vi "varshni fit function.vi"(3 "output control":T1, 4 "data":T2, 5 "X":dbl[](array[numeric]), 6 "a":dbl[](array[numeric])) -> (0 "error out":errorcluster, 1 "f'(X,a)":dbl[][](array[numeric]), 2 "f(X,a)":dbl[](array[numeric]))   [LabVIEW 2010]
doc: "This template is the starting point for creating a model function to be passed to the Nonlinear Curve Fit.vi."
uses:
  <vilib>/gmath/NumericalOptimization/objective function data.ctl
  <vilib>/gmath/NumericalOptimization/LM_output select.ctl
  <vilib>/gmath/NI_Gmath.lvlib
panel:
  in  "fit":enum16{"other", "3par", "5par"}(ring)=enum."3par"
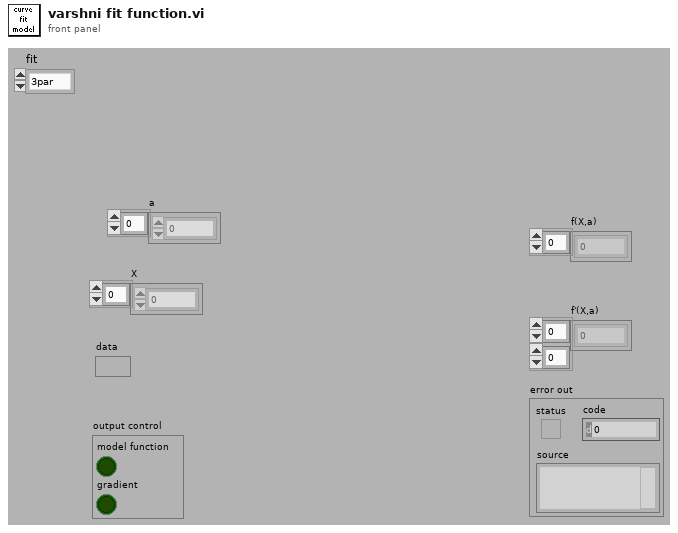
[diagram p1: front panel]
types:
  T1 = typedef "NI_Gmath.lvlib/LM_output select.ctl" = cluster{"model function":bool, "gradient":bool}
  T2 = typedef "NI_Gmath.lvlib/objective function data.ctl" = variant
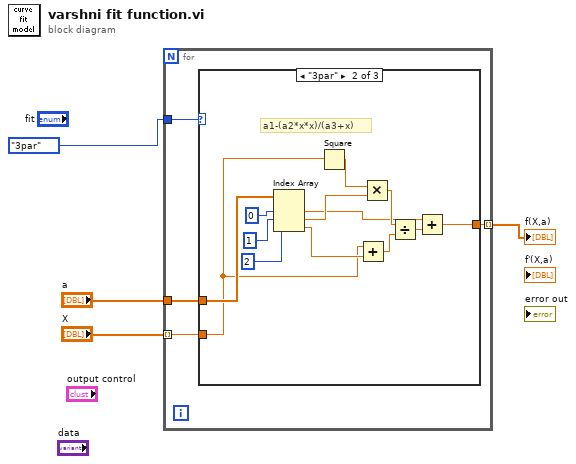
[diagram p0: block diagram]
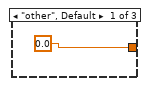
[diagram p2: hidden frame]
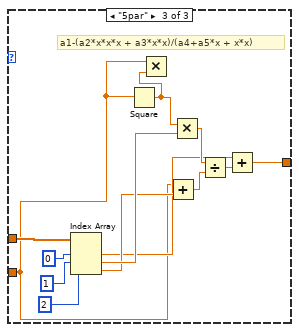
[diagram p3: hidden frame]
diagram:
  n1 = for {
    tunnel: "a" -> [w8]
    tunnel: "X" -> [w6] mode=indexing
    tunnel: [w7] -> w2 mode=indexing
    tunnel: enum16{"other", "3par", "5par"}."3par" ("action") -> [w5]
    n2 = case shown="\"3par\"" w5 {
      tunnel: w8 -> [_ w22 w35]
      tunnel: [0.0 w12 w25] -> w7
      tunnel: w6 -> [_ w11 w24]
      frame "other", Default {
      }
      frame "3par" {
        # "a1-(a2*x*x)/(a3+x)"
        n3 = Index Array(array=w22, index #1=0 ("index"), index #2=1 ("index"), index #3=2 ("index")) -> (element #1=w14:dbl, element #2=w18:dbl, element #3=w17:dbl)
        n4 = Square(x=w11) -> (x^2=w10:dbl)
        n5 = Add(x=w11, y=w17) -> (x+y=w15:dbl)
        n6 = Multiply(x=w10, y=w18) -> (x*y=w16:dbl)
        n7 = Divide(x=w16, y=w15) -> (x/y=w13:dbl)
        n8 = Add(x=w14, y=w13) -> (x+y=w12:dbl)
      }
      frame "5par" {
        # "a1-(a2*x*x*x + a3*x*x)/(a4+a5*x + x*x)"
        n9 = Index Array(array=w35, index #1=0 ("index"), index #2=1 ("index"), index #3=2 ("index")) -> (element #1=w27:dbl, element #2=w31:dbl, element #3=w30:dbl)
        n10 = Square(x=w24) -> (x^2=w23:dbl)
        n11 = Multiply(x=w24, y=w23) -> ()  [unwired: 1 out]
        n12 = Add(x=w24, y=w30) -> (x+y=w28:dbl)
        n13 = Multiply(x=w23, y=w31) -> (x*y=w29:dbl)
        n14 = Divide(x=w29, y=w28) -> (x/y=w26:dbl)
        n15 = Add(x=w27, y=w26) -> (x+y=w25:dbl)
      }
    }
  }
  "f(X,a)" <- w2
